vi "Query Lock.vi"(8 "error in (no error)":errorcluster, 10 "Motor ID (0)":u8, 11 "Dynamixel Motor VISA in":refnum<class "Dynamixel Motor VISA.lvclass">) -> (0 "error out":errorcluster, 2 "EEPROM Locked":bool, 3 "Dynamixel Motor VISA out":refnum<class "Dynamixel Motor VISA.lvclass">)   [LabVIEW 2016, in "Dynamixel Motor VISA.lvclass"]
doc: "Checks to see if the motor has been locked. If it has been locked, then addresses in the EEPROM (0-23) cannot be modified until the motor's power is cycled."
uses:
  <instrlib>/Dynamixel Motor/HAIOL/VISA/Dynamixel Motor VISA.lvclass
  <instrlib>/Dynamixel Motor/HAIOL/VISA/Dynamixel Motor VISA.lvclass/Dynamixel Motor VISA.ctl
  <instrlib>/Dynamixel Motor/Dynamixel Motor.lvlib
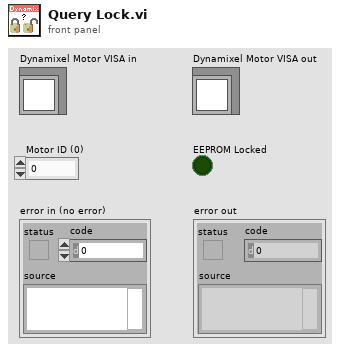
[diagram p1: front panel]
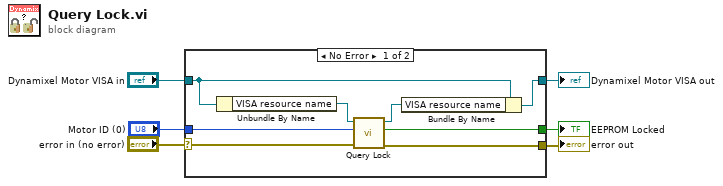
[diagram p0: block diagram]
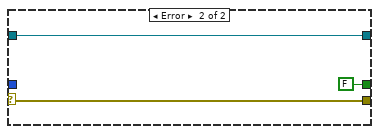
[diagram p2: hidden frame]
diagram:
  n1 = case shown="No Error" "error in (no error)" {
    selector: "error in (no error)" -> [w14 w15]
    tunnel: "Dynamixel Motor VISA in" -> [w10 w17]
    tunnel: "Motor ID (0)" -> [w12 _]
    tunnel: [w11 w15] -> w3
    tunnel: [w8 w17] -> w2
    tunnel: [w7 FALSE ("EEPROM Locked")] -> w1
    frame No Error {
      n2 = Unbundle By Name(w10) -> ("VISA resource name"=w13:refnum<visa-resource-name>)
      n3 = call <instrlib>:"Query Lock.vi"("error in (no error)"=w14, "Motor ID (0)"=w12, "VISA resource name"=w13) -> ("error out"=w11:errorcluster, "EEPROM Locked"=w7:bool, "VISA resource name out"=w9:refnum<visa-resource-name>)  [unwired: 6 in]
      n4 = Bundle By Name(cluster=w10, "VISA resource name"=w9) -> (w8:refnum<class "Dynamixel Motor VISA.lvclass">)
    }
    frame Error {
    }
  }
  "error out" <- w3
  "Dynamixel Motor VISA out" <- w2
  "EEPROM Locked" <- w1
